vi "Mechanum.vi"   [LabVIEW 2012]
uses:
  <vilib>/NXT/Block Support/NXT_OutputPort.ctl
  <vilib>/NXT/Dual Mode Library/Waits/Wait_Num.vi
  <vilib>/NXT/NXTIO Xnodes/NXTIONodeSubVIs/NXTMoveMotors.vi
  <vilib>/NXT/Subs/LVHSConnector.ctl
  <vilib>/NXT/NXTIO Xnodes/AddressXNode/NXTIOAddress.xnode
  <vilib>/NXT/NXTIO Xnodes/NXTIOXNode/NXTIO.xnode
  <vilib>/NXT/LegoClasses/BrickReference/BrickReference.lvclass
types:
  T1 = typedef "NXT_OutputPort.ctl" = u8
  T2 = cluster{"Output Port":T1, "Output Port 2":T1, "Output Port 3":T1, "Output Port 4":T1}
  T3 = cluster{"Port":T1, "Port":T1, "Port":T1, "Port":T1}
  T4 = typedef "LVHSConnector.ctl" = refnum<class "BrickReference.lvclass">
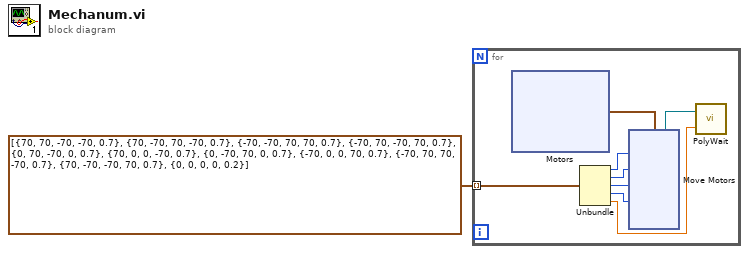
[diagram p0: block diagram]
diagram:
  n1 = for {
    tunnel: cluster{i32, i32, i32, i32, dbl}[] [{70, 70, -70, -70, 0.7}, {70, -70, 70, -70, 0.7}, {-70, -70, 70, 70, 0.7}, {-70, 70, -70, 70, 0.7}, {0, 70, -70, 0, 0.7}, {70, 0, 0, -70, 0.7}, {0, -70, 70, 0, 0.7}, {-70, 0, 0, 70, 0.7}, {-70, 70, 70, -70, 0.7}, {70, -70, -70, 70, 0.7}, {0, 0, 0, 0, 0.2}] -> [w8] mode=indexing
    n2 = xnode "Motors"() -> ("Motor"=w9:T3)
    n3 = Unbundle(w8) -> (w7:i32, w6:i32, w5:i32, w4:i32, w3:dbl)
    n4 = xnode "Move Motors"("Power/Speed 4"=w4, "Power/Speed 3"=w5, "Power/Speed 2"=w6, "Power/Speed 1"=w7, "Motors"=w9) -> ("NXT/EV3"=w2:T4)  [unwired: 1 in]
    n5 = call-poly <vilib>:"PolyWait.vi"("Time (1 sec)"=w3, "NXT/EV3"=w2) -> ()  [unwired: 2 in, 1 out]
  }
